vi "RP set frequency batch.vi"(8 "Error In":errorcluster, 10 "Frequency":dbl[](array[numeric]), 11 "connection ID":refnum<k5>) -> (0 "Error Out":errorcluster, 2 "Phase words sent":u32[](array[numeric]), 3 "connection ID out":refnum<k5>)   [LabVIEW 2015]
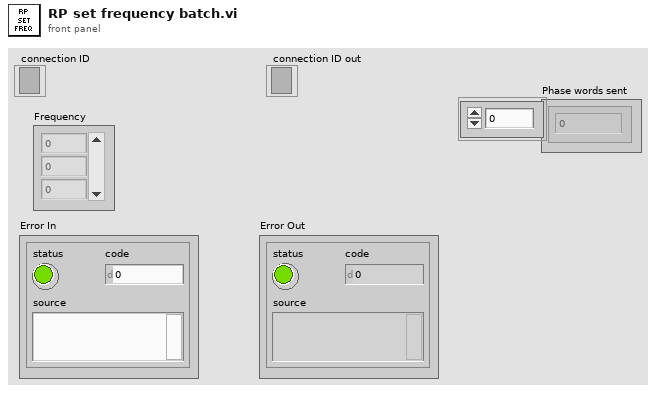
[diagram p1: front panel]
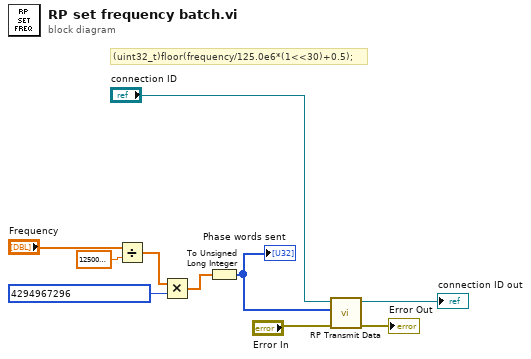
[diagram p0: block diagram]
diagram:
  # "(uint32_t)floor(frequency/125.0e6*(1<<30)+0.5);"
  n1 = Divide(x="Frequency", y=125000000.0) -> (x/y=w8:dbl[])
  n2 = Multiply(x=w8, y=i64 4294967296) -> (x*y=w7:dbl[])
  n3 = To Unsigned Long Integer(number=w7) -> (unsigned 32bit integer=w4:u32[])
  "Phase words sent" <- w4
  n4 = call "RP Transmit Data.vi"("Error In"="Error In", "Data"=w4, "connection ID"="connection ID") -> ("Error Out"=→"Error Out":errorcluster, "connection ID out"=→"connection ID out":refnum<k5>)  [unwired: 7 in]
